vi "CSM MDI Example.vi"   [LabVIEW 2020, in "MDI ViewManager.lvlib"]
uses:
  MDI ViewManager.lvlib
  Typedef/UpdateInsertableVICtl.ctl
  b95e2d39-9a72-4fb7-b733-c53d2ceefbbe.vi
  8616cbc6-d8ba-435f-9af2-03ccb79b2d5e.vi
  <userlib>/_NEVSTOP/Communicable State Machine(CSM)/_Polymophic/Build No-Reply Asynchronous Message with Arguments.vi
  <userlib>/_NEVSTOP/Communicable State Machine(CSM)/addons/API-String-Arugments-Support/_Support/Data To API String Arguments.vi
  <userlib>/_NEVSTOP/Communicable State Machine(CSM)/Communicable State Machine.lvlib
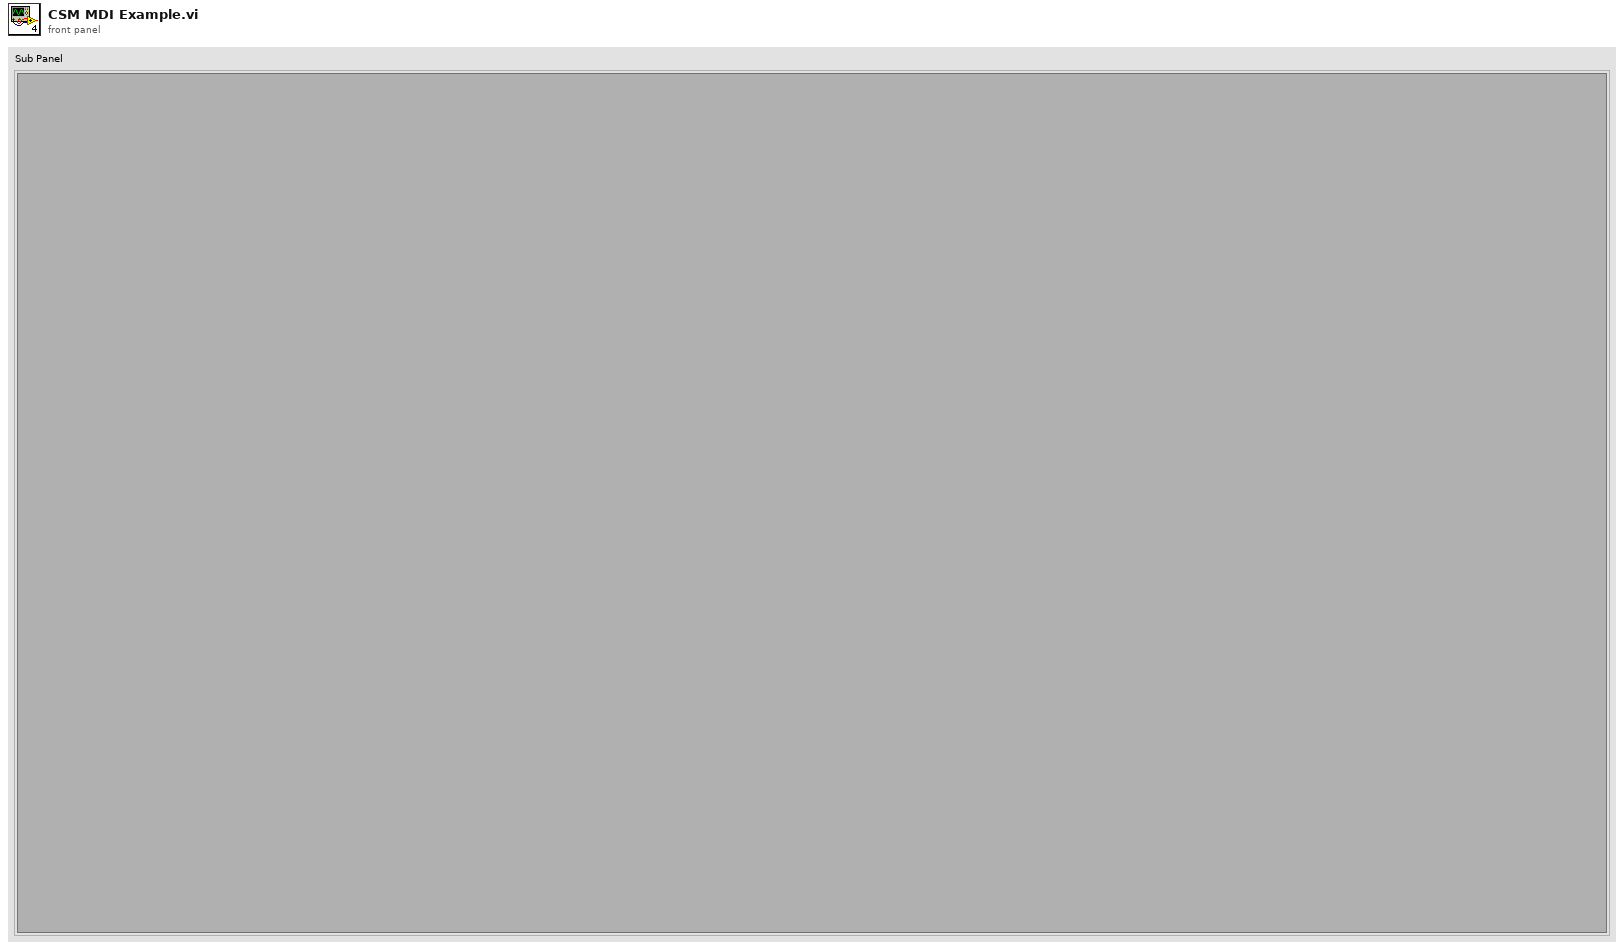
[diagram p1: front panel]
types:
  T1 = typedef "MDI ViewManager.lvlib/UpdateInsertableVICtl.ctl" = cluster{"Name":string, "VIPath":path, "Height(Default)":dbl, "Widht(Default)":dbl}
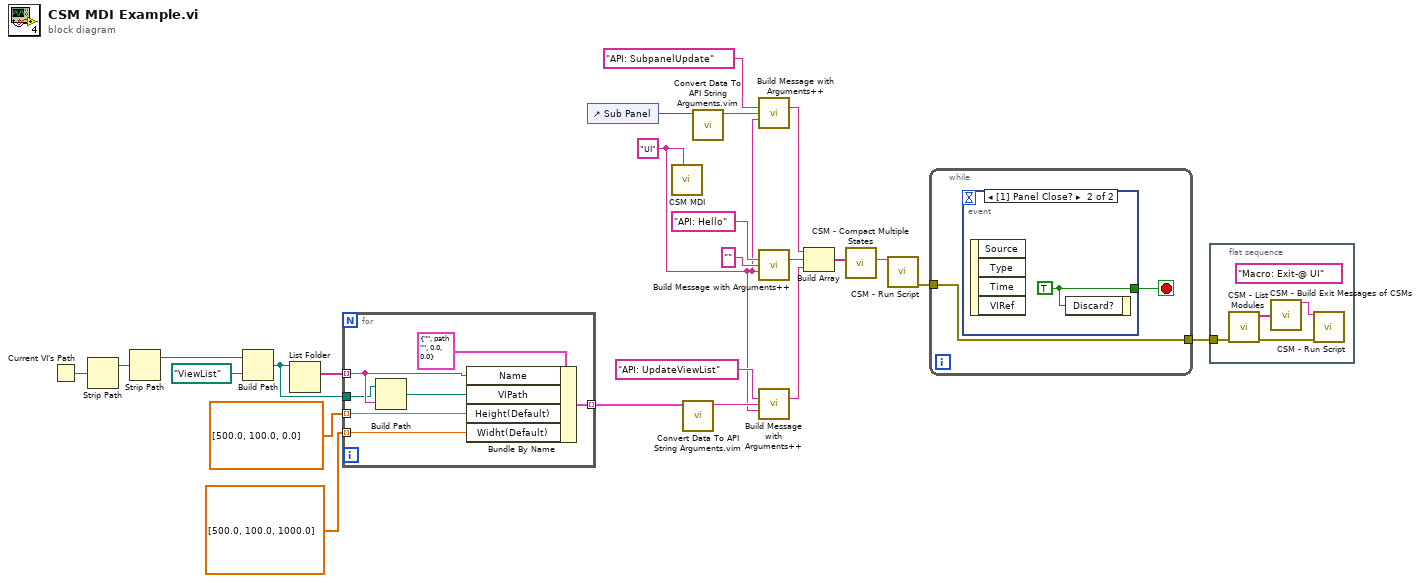
[diagram p0: block diagram]
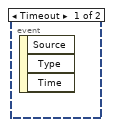
[diagram p2: hidden frame]
diagram:
  w8 = "UI" ("Name (\"\" to Use UUID)")
  n1 = Current VI's Path() -> (path=w7:path)
  n2 = Strip Path(path=w7) -> (stripped path=w4:path)  [unwired: 1 out]
  n3 = Strip Path(path=w4) -> (stripped path=w3:path)  [unwired: 1 out]
  n4 = Build Path(base path=w3, name or relative path=path "ViewList" ("path")) -> (appended path=w5:path)
  n5 = List Folder(path=w5) -> (filenames=w14:string[])  [unwired: 3 in, 3 out]
  n6 = for {
    tunnel: w14 -> [w30] mode=indexing
    tunnel: w5 -> [w29]
    tunnel: [w27] -> w13 mode=indexing
    tunnel: dbl[] [500.0, 100.0, 1000.0] ("Widht(Default)") -> [w26] mode=indexing
    tunnel: dbl[] [500.0, 100.0, 0.0] ("Height(Default)") -> [w25] mode=indexing
    n7 = Build Path(base path=w29, name or relative path=w30) -> (appended path=w28:path)
    n8 = Bundle By Name(cluster=T1 {"Name"="", "VIPath"=path "", "Height(Default)"=0.0, "Widht(Default)"=0.0} ("Array"), "Name"=w30, "VIPath"=w28, "Height(Default)"=w25, "Widht(Default)"=w26) -> (w27:T1)
  }
  n9 = control-ref of="Sub Panel"() -> (w22:refnum<vi>)
  n10 = call "CSM MDI.vi"("Name (\"\" to Use UUID)"=w8) -> ()  [unwired: 11 in]
  n11 = call "Convert Data To API String Arguments.vim"("Data"=w13) -> ("API String"=w12:string)  [unwired: 7 in, 1 out]
  n12 = call "Convert Data To API String Arguments.vim"("Data"=w22) -> ("API String"=w21:string)  [unwired: 7 in, 1 out]
  n13 = call-poly <userlib>:"Build Message with Arguments++.vi"("State With Arguments"="API: SubpanelUpdate", "Arguments (\"\")"=w21, "Target Module (\"\")"=w8) -> ("CSM Message String"=w20:string)  [unwired: 12 in]
  n14 = call-poly <userlib>:"Build Message with Arguments++.vi"("State With Arguments"="API: Hello", "Arguments (\"\")"="" ("Arguments (\"\")"), "Target Module (\"\")"=w8) -> ("CSM Message String"=w18:string)  [unwired: 12 in]
  n15 = call-poly <userlib>:"Build Message with Arguments++.vi"("State With Arguments"="API: UpdateViewList", "Arguments (\"\")"=w12, "Target Module (\"\")"=w8) -> ("CSM Message String"=w10:string)  [unwired: 12 in]
  n16 = Build Array(w20, w18, w10) -> (w17:string[])
  n17 = call <userlib>:"CSM - Compact Multiple States.vi"("Multiple States"=w17) -> ("States"=w16:string)  [unwired: 9 in]
  n18 = call <userlib>:"CSM - Run Script.vi"("CSM Scripts"=w16) -> ("error out"=w24:errorcluster)  [unwired: 12 in, 2 out]
  n19 = while {
    tunnel: w24 -> [w32]
    tunnel: [w32] -> w9
    stop <- w33 stop-if-true
    n20 = event shown="[1] Panel Close?" {
      selector: _ -> [_ _]
      dyn-events: _ -> [_ _]
      timeout: _ -> [_ _]
      tunnel: [_ w34] -> w33
      event Timeout {
        n21 = event-data() -> ()  [unwired: 1 in, 3 out]
      }
      event Panel Close? {
        w34 = TRUE ("Discard?")
        n22 = event-data() -> ()  [unwired: 1 in, 4 out]
        n23 = event-data("Discard?"=w34) -> ()  [unwired: 1 in, 1 out]
      }
    }
  }
  n24 = flat-sequence {
    tunnel: w9 -> [w37]
    frame #0 {
      (unwired) "Macro: Exit-@ UI" ("CSM Scripts")
      n25 = call <userlib>:"CSM - List Modules.vi"("Error In"=w37) -> ("error out"=w35:errorcluster, "Module Names"=w38:string[])  [unwired: 9 in]
      n26 = call <userlib>:"CSM - Build Exit Messages of CSMs.vi"("CSMs"=w38) -> ("States"=w36:string)  [unwired: 14 in]
      n27 = call <userlib>:"CSM - Run Script.vi"("CSM Scripts"=w36, "error in (no error)"=w35) -> ()  [unwired: 11 in, 3 out]
    }
  }
